vi "2B Dizinin Ortalama Değeri.vi"() -> ()   [LabVIEW 2014]
panel:
  out "Toplam":dbl
  out "Aritmetik Ortalama":dbl
  in  "Array":dbl[][](array[numeric])
  # "3x3'lük dizinin elelmanlarının aritmetik ortalamasını\nhesaplayanprogramı yazınız."
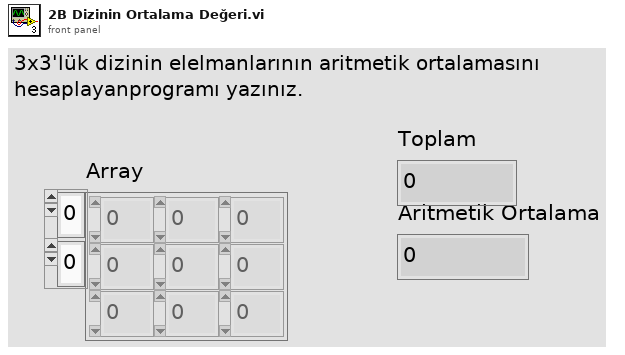
[diagram p1: front panel]
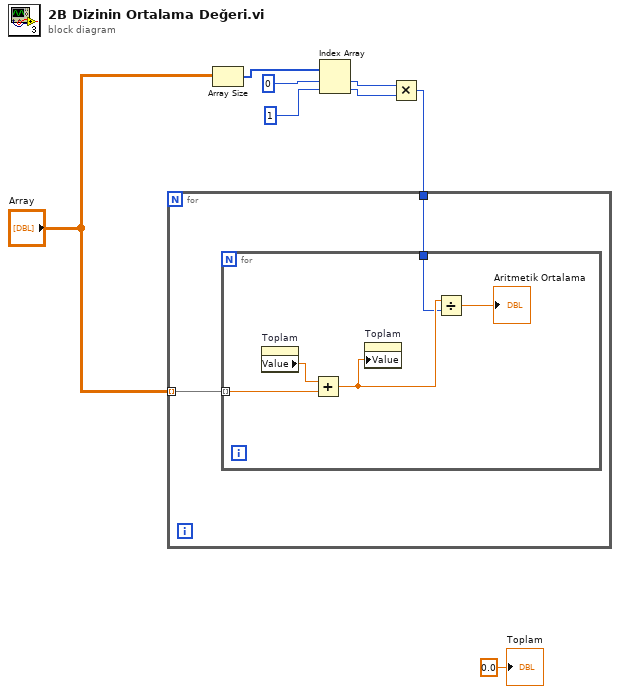
[diagram p0: block diagram]
diagram:
  n1 = Array Size(array="Array") -> (size(s)=w8:i32[])
  n2 = Index Array(array=w8, index #1=0 ("index"), index #2=1 ("index")) -> (element #1=w4:i32, element #2=w5:i32)
  n3 = Multiply(x=w4, y=w5) -> (x*y=w1:i32)
  n4 = for {
    tunnel: "Array" -> [w10] mode=indexing
    tunnel: w1 -> [w9]
    n5 = for {
      tunnel: w10 -> [w14] mode=indexing
      tunnel: w9 -> [w11]
      n6 = property on="Toplam" class="DigNum (strict)"() -> ("Value"=w15:dbl)  [unwired: 2 in, 2 out]
      n7 = Add(x=w15, y=w14) -> (x+y=w12:dbl)
      n8 = property on="Toplam" class="DigNum (strict)"("Value"=w12) -> ()  [unwired: 2 in, 2 out]
      n9 = Divide(x=w12, y=w11) -> (x/y=→"Aritmetik Ortalama":dbl)
    }
  }
  "Toplam" <- 0.0 ("Toplam")
